vi "Set RowNumDisplay.vi"(8 "error in (no error)":errorcluster, 10 "RowNumDisplay":u16, 11 "Multicolumn ListBox in":refnum<class "Multicolumn ListBox.lvclass">) -> (0 "error out":errorcluster, 3 "Multicolumn ListBox out":refnum<class "Multicolumn ListBox.lvclass">)   [LabVIEW 2018, in "Multicolumn ListBox.lvclass"]
uses:
  Multicolumn ListBox.lvclass
  Multicolumn ListBox.lvclass/Multicolumn ListBox.ctl
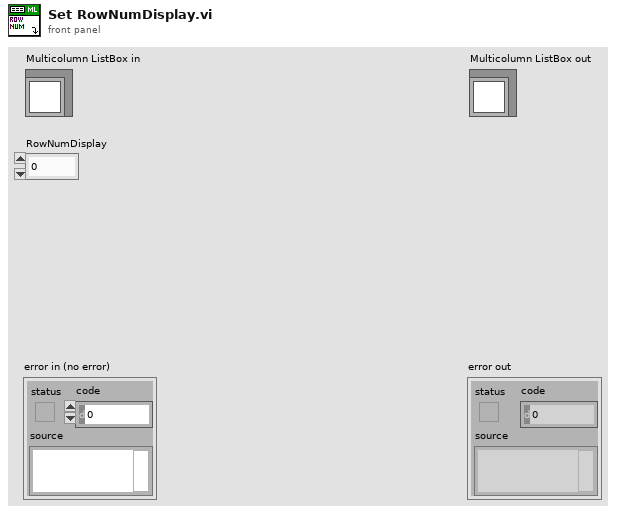
[diagram p1: front panel]
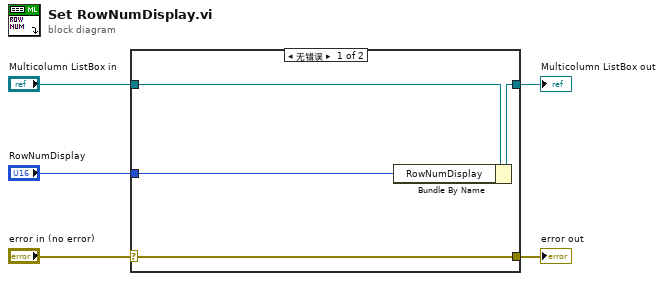
[diagram p0: block diagram]
diagram:
  n1 = case shown="无错误" "error in (no error)" {
    selector: "error in (no error)" -> [w9 w10]
    tunnel: [w9 w10] -> w4
    tunnel: [w7 w11] -> w2
    tunnel: "Multicolumn ListBox in" -> [w8 w11]
    tunnel: "RowNumDisplay" -> [w6 _]
    frame No Error {
      n2 = Bundle By Name(cluster=w8, "RowNumDisplay"=w6) -> (w7:refnum<class "Multicolumn ListBox.lvclass">)
    }
    frame Error {
    }
  }
  "error out" <- w4
  "Multicolumn ListBox out" <- w2
